vi "zapis.vi"() -> ()   [LabVIEW 2020]
panel:
  out "Flow":dbl
  out "Turbidity":dbl
  out "Temperature":dbl
  out "Substrate dosing":bool
  out "Redox":dbl
  out "Recycle":bool
  out "pH":dbl
  out "Oxygen":dbl
  out "Overflow":bool
  out "Mixing [%]":dbl
  out "Mixer":bool
  out "Feed":bool
  out "CO2":dbl
  out "Aeration":bool
  out "Level":dbl
  in  "Stop Button":bool
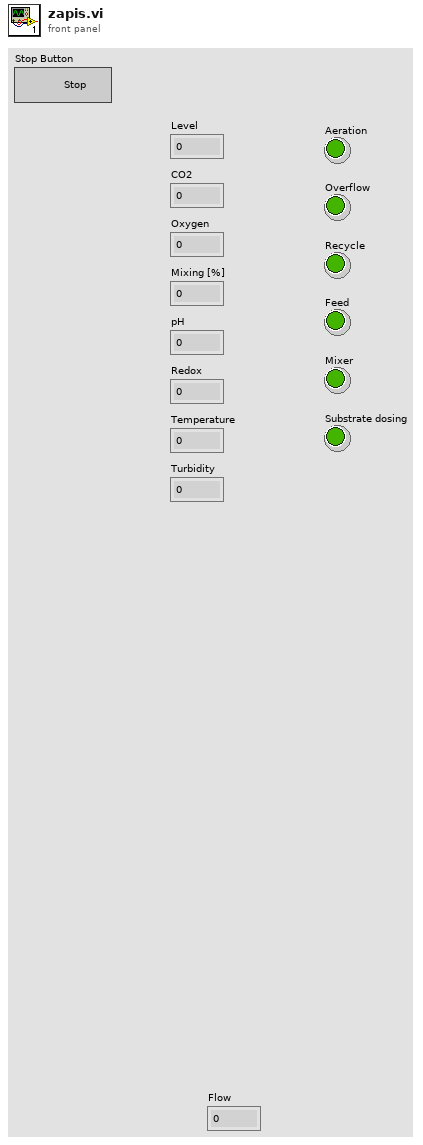
[diagram p1: front panel]
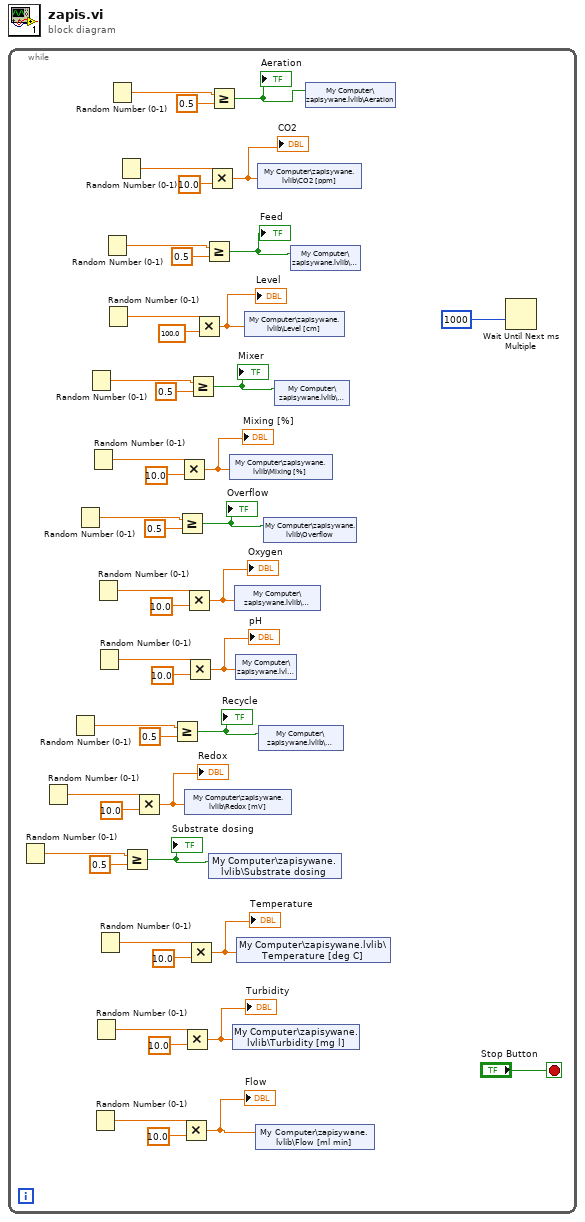
[diagram p0: block diagram]
diagram:
  n1 = while {
    stop <- "Stop Button" stop-if-true
    n2 = Random Number (0-1)() -> (number: 0 to 1=w12:dbl)
    n3 = Random Number (0-1)() -> (number: 0 to 1=w15:dbl)
    n4 = Random Number (0-1)() -> (number: 0 to 1=w18:dbl)
    n5 = Random Number (0-1)() -> (number: 0 to 1=w27:dbl)
    n6 = Random Number (0-1)() -> (number: 0 to 1=w33:dbl)
    n7 = Random Number (0-1)() -> (number: 0 to 1=w30:dbl)
    n8 = Random Number (0-1)() -> (number: 0 to 1=w3:dbl)
    n9 = Random Number (0-1)() -> (number: 0 to 1=w6:dbl)
    n10 = Random Number (0-1)() -> (number: 0 to 1=w24:dbl)
    n11 = Random Number (0-1)() -> (number: 0 to 1=w21:dbl)
    n12 = Random Number (0-1)() -> (number: 0 to 1=w9:dbl)
    n13 = Random Number (0-1)() -> (number: 0 to 1=w36:dbl)
    n14 = Random Number (0-1)() -> (number: 0 to 1=w45:dbl)
    n15 = Random Number (0-1)() -> (number: 0 to 1=w42:dbl)
    n16 = Random Number (0-1)() -> (number: 0 to 1=w39:dbl)
    n17 = Greater Or Equal?(x=w12, y=0.5) -> (x >= y?=w10:bool)
    "Substrate dosing" <- w10
    n18 = Multiply(x=w15, y=10.0) -> (x*y=w13:dbl)
    "Redox" <- w13
    n19 = Greater Or Equal?(x=w18, y=0.5) -> (x >= y?=w16:bool)
    "Recycle" <- w16
    n20 = Greater Or Equal?(x=w27, y=0.5) -> (x >= y?=w25:bool)
    "Overflow" <- w25
    n21 = Multiply(x=w30, y=10.0) -> (x*y=w28:dbl)
    "Mixing [%]" <- w28
    n22 = Multiply(x=w3, y=10.0) -> (x*y=w1:dbl)
    "Flow" <- w1
    n23 = Multiply(x=w6, y=10.0) -> (x*y=w4:dbl)
    "Turbidity" <- w4
    n24 = Multiply(x=w24, y=10.0) -> (x*y=w22:dbl)
    "Oxygen" <- w22
    n25 = Multiply(x=w21, y=10.0) -> (x*y=w19:dbl)
    "pH" <- w19
    n26 = shared-variable "My Computer\\zapisywane.lvlib\\Redox [mV]"(w13) -> ()  [unwired: 1 in, 1 out]
    n27 = Multiply(x=w9, y=10.0) -> (x*y=w7:dbl)
    "Temperature" <- w7
    n28 = Greater Or Equal?(x=w33, y=0.5) -> (x >= y?=w31:bool)
    "Mixer" <- w31
    n29 = Multiply(x=w45, y=100.0) -> (x*y=w43:dbl)
    "Level" <- w43
    n30 = Greater Or Equal?(x=w36, y=0.5) -> (x >= y?=w34:bool)
    "Feed" <- w34
    n31 = Multiply(x=w39, y=10.0) -> (x*y=w37:dbl)
    "CO2" <- w37
    n32 = Greater Or Equal?(x=w42, y=0.5) -> (x >= y?=w40:bool)
    "Aeration" <- w40
    n33 = shared-variable "My Computer\\zapisywane.lvlib\\Substrate dosing"(w10) -> ()  [unwired: 1 in, 1 out]
    n34 = shared-variable "My Computer\\zapisywane.lvlib\\Mixing [%]"(w28) -> ()  [unwired: 1 in, 1 out]
    n35 = shared-variable "My Computer\\zapisywane.lvlib\\Turbidity [mg l]"(w4) -> ()  [unwired: 1 in, 1 out]
    n36 = shared-variable "My Computer\\zapisywane.lvlib\\Oxygen"(w22) -> ()  [unwired: 1 in, 1 out]
    n37 = shared-variable "My Computer\\zapisywane.lvlib\\pH"(w19) -> ()  [unwired: 1 in, 1 out]
    n38 = shared-variable "My Computer\\zapisywane.lvlib\\Temperature [deg C]"(w7) -> ()  [unwired: 1 in, 1 out]
    n39 = shared-variable "My Computer\\zapisywane.lvlib\\Level [cm]"(w43) -> ()  [unwired: 1 in, 1 out]
    n40 = shared-variable "My Computer\\zapisywane.lvlib\\Flow [ml min]"(w1) -> ()  [unwired: 1 in, 1 out]
    n41 = shared-variable "My Computer\\zapisywane.lvlib\\CO2 [ppm]"(w37) -> ()  [unwired: 1 in, 1 out]
    n42 = shared-variable "My Computer\\zapisywane.lvlib\\Recycle"(w16) -> ()  [unwired: 1 in, 1 out]
    n43 = shared-variable "My Computer\\zapisywane.lvlib\\Overflow"(w25) -> ()  [unwired: 1 in, 1 out]
    n44 = shared-variable "My Computer\\zapisywane.lvlib\\Mixer"(w31) -> ()  [unwired: 1 in, 1 out]
    n45 = shared-variable "My Computer\\zapisywane.lvlib\\Feed"(w34) -> ()  [unwired: 1 in, 1 out]
    n46 = shared-variable "My Computer\\zapisywane.lvlib\\Aeration"(w40) -> ()  [unwired: 1 in, 1 out]
    n47 = Wait Until Next ms Multiple(millisecond multiple=u32 1000) -> ()  [unwired: 1 out]
  }
